vi "Detect Barcodes (ARGB).vi"(8 "error in (no error)":errorcluster, 10 "ARGB Image":T4, 11 "Barcode Detector in":refnum<class "Barcode Detector.lvclass">) -> (0 "error out":errorcluster, 2 "Detections":T1[](array[typedef]), 3 "Barcode Detector (Duplicate)":refnum<class "Barcode Detector.lvclass">)   [LabVIEW 2020, in "g_ar_toolkit.feature_detection.lvlib" / "Barcode Detector.lvclass"]
uses:
  Barcode Detector.lvclass
  g_ar_toolkit.image/ARGB Image.ctl
  Detection.ctl
  Detection Region.ctl
  g_ar_toolkit.common/Image Point (Integer).ctl
  Barcode Detector.lvclass/Barcode Detector.ctl
  5cbfdd98-1063-43fc-ab47-121d1b6d8619.vi
  g_ar_toolkit.common/Module Path.vi
  <vilib>/Utility/error.llb/Error Cluster From Error Code.vi
  g_ar_toolkit.common/g_ar_toolkit.common.lvlib
  g_ar_toolkit.image/g_ar_toolkit.image.lvlib
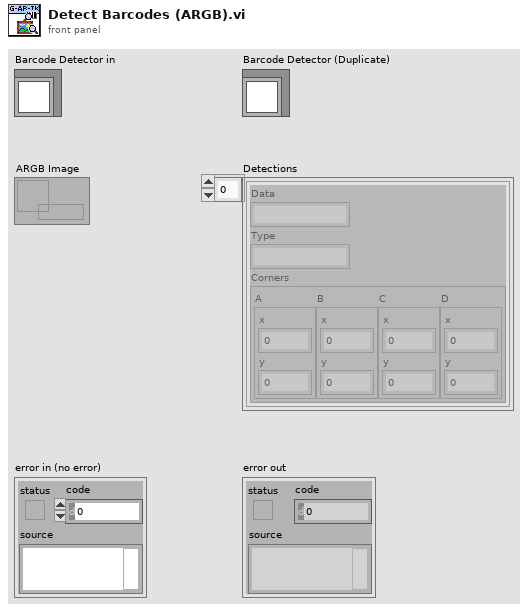
[diagram p1: front panel]
types:
  T1 = typedef "g_ar_toolkit.feature_detection.lvlib/Barcode Detector.lvclass/Detection.ctl" = cluster{"Data":string, "Type":string, "Corners":T2}
  T2 = typedef "g_ar_toolkit.feature_detection.lvlib/Barcode Detector.lvclass/Detection Region.ctl" = cluster{"A":T3, "B":T3, "C":T3, "D":T3}
  T3 = typedef "g_ar_toolkit.common.lvlib/Image Point (Integer).ctl" = cluster{"x":i32, "y":i32}
  T4 = typedef "g_ar_toolkit.image.lvlib/ARGB Image.ctl" = refnum<data-value>
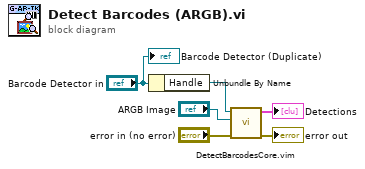
[diagram p0: block diagram]
diagram:
  n1 = Unbundle By Name("Barcode Detector in") -> ("Handle"=w1:refnum<data-value>)
  n2 = call "DetectBarcodesCore.vim"("error in (no error)"="error in (no error)", "Greyscale Image"="ARGB Image", "Handle"=w1) -> ("error out"=→"error out":errorcluster, "Detections"=→"Detections":T1[])  [unwired: 7 in]
  "Barcode Detector (Duplicate)" <- "Barcode Detector in"
